vi "HasAllSamples.vi"(8 "error in (no error)":errorcluster, 11 "Automation in":refnum<class "Automation.lvclass">) -> (0 "error out":errorcluster, 2 "Has all samples?":bool, 3 "Automation out":refnum<class "Automation.lvclass">)   [LabVIEW 2019]
uses:
  Automation.lvclass
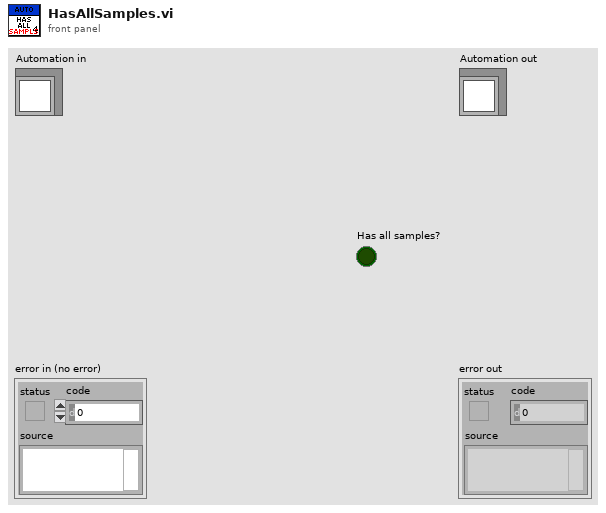
[diagram p1: front panel]
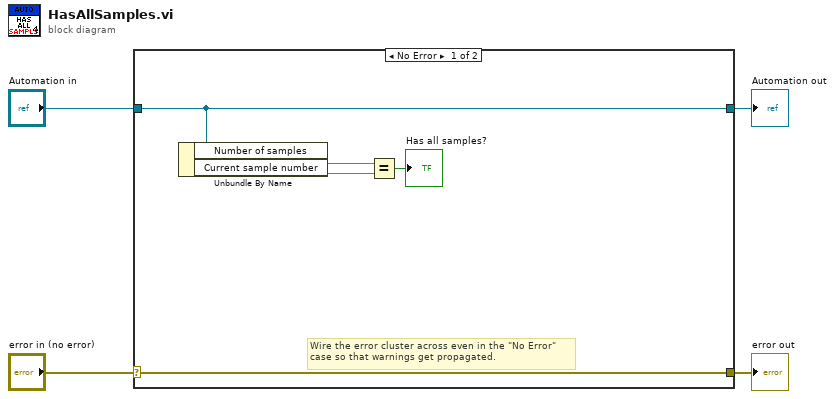
[diagram p0: block diagram]
diagram:
  n1 = case shown="No Error" "error in (no error)" {
    selector: "error in (no error)" -> [w9 w11]
    tunnel: [w9 w11] -> w3
    tunnel: [w8 w10] -> w1
    tunnel: "Automation in" -> [w8 w10]
    frame No Error {
      # "Wire the error cluster across even in the \"No Error\"\ncase so that warnings get propagated."
      n2 = Unbundle By Name(w8) -> ("Number of samples"=w5, "Current sample number"=w6)
      n3 = Equal?(x=w5, y=w6) -> (x = y?=→"Has all samples?":bool)
    }
    frame Error {
    }
  }
  "error out" <- w3
  "Automation out" <- w1
